vi "SteeringFrameV_To_MotorV(SubVI).vi"(11 "Steering frame velocities":dbl[](array[numeric])) -> (2 "right_motor_velocity":dbl, 3 "Left_motor_velocity":dbl)   [LabVIEW 2017]
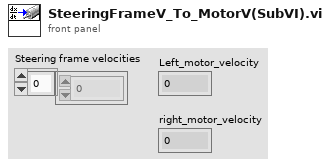
[diagram p1: front panel]
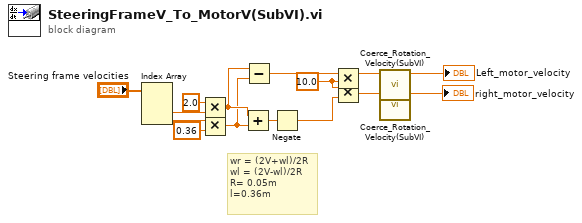
[diagram p0: block diagram]
diagram:
  w2 = 10.0 ("y")
  # "wr = (2V+wl)/2R\nwl = (2V-wl)/2R\nR= 0.05m\nl=0.36m"
  n1 = Index Array(array="Steering frame velocities") -> (element #2=w8:dbl, element #3=w10:dbl)  [unwired: 3 in, 1 out]
  n2 = Multiply(x=2.0, y=w8) -> (x*y=w14:dbl)
  n3 = Multiply(x=w10, y=0.36) -> (x*y=w13:dbl)
  n4 = Add(x=w14, y=w13) -> (x+y=w15:dbl)
  n5 = Subtract(x=w14, y=w13) -> (x-y=w12:dbl)
  n6 = Negate(x=w15) -> (-x=w1:dbl)
  n7 = Multiply(x=w12, y=w2) -> (x*y=w4:dbl)
  n8 = Multiply(x=w2, y=w1) -> (x*y=w3:dbl)
  n9 = call "Coerce_Rotation_Velocity(SubVI).vi"("Rotation_velocity_in"=w4) -> ("Rotation_velocity_out"=→"Left_motor_velocity":dbl)  [unwired: 10 in]
  n10 = call "Coerce_Rotation_Velocity(SubVI).vi"("Rotation_velocity_in"=w3) -> ("Rotation_velocity_out"=→"right_motor_velocity":dbl)  [unwired: 10 in]
